vi "PIM Strip-Chart.vi"(4 "Clear Buffer (f)":bool, 5 "Buffer Length (2048)":i32=2048, 6 "Update Time, sec":dbl format="%.2f", 7 "Measured Values":dbl[](array[numeric])) -> (3 "Traces":cluster{"x-values":dbl[], "y-values":dbl[]}[](array[cluster]) {"y-values" format="%.2f"; "x-values" format="%.2f"})   [LabVIEW 2011]
doc: "Accepts a five element cluster of data points and buffers these into five separate clusters within an array (suitable for passing to an XY Chart).\n\nThe time, in Seconds since last reset, is placed in the x-value array for each line on the plot."
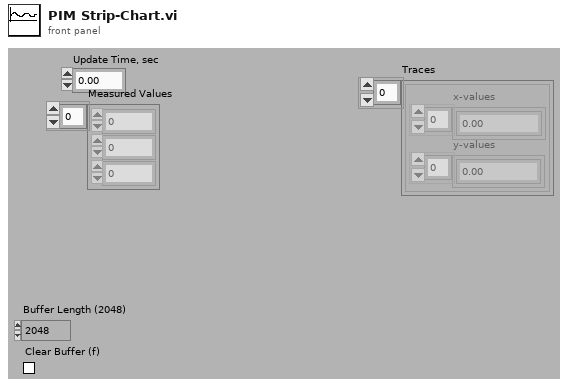
[diagram p1: front panel]
types:
  T1 = cluster{"Measured Values[0]":dbl, "Measured Values[1]":dbl}
  T2 = cluster{"Measured Values[0]":dbl, "Measured Values[1]":dbl, "Measured Values[2]":dbl, "Measured Values[3]":dbl, "Measured Values[4]":dbl}
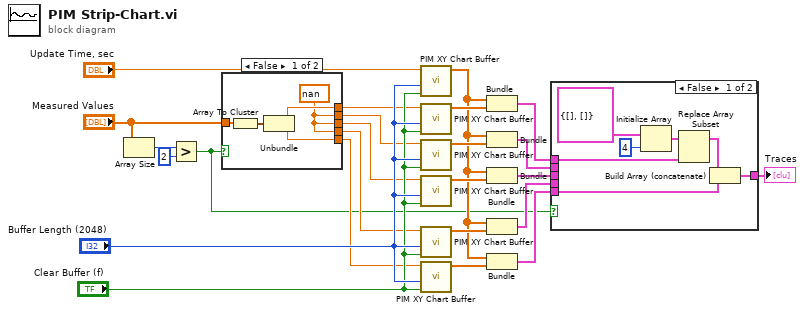
[diagram p0: block diagram]
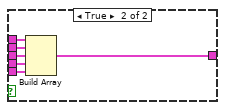
[diagram p2: hidden frame]
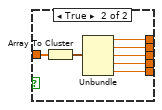
[diagram p3: hidden frame]
diagram:
  n1 = Array Size(array="Measured Values") -> (size(s)=w20:i32)
  n2 = Greater?(x=w20, y=2) -> (0:w1:bool)
  n3 = case shown="False" w1 {
    tunnel: "Measured Values" -> [w28 w36]
    tunnel: [w27 w35] -> w11
    tunnel: [w25 w34] -> w9
    tunnel: [w25 w33] -> w8
    tunnel: [w25 w32] -> w7
    tunnel: [w26 w31] -> w6
    frame False {
      w25 = nan ("Measured Values[3]")
      n4 = Array To Cluster(array=w28) -> (cluster=w29:T1)
      n5 = Unbundle(w29) -> ("Measured Values[0]"=w27:dbl, "Measured Values[1]"=w26:dbl)
    }
    frame True {
      n6 = Array To Cluster(array=w36) -> (cluster=w30:T2)
      n7 = Unbundle(w30) -> ("Measured Values[0]"=w35:dbl, "Measured Values[1]"=w34:dbl, "Measured Values[2]"=w33:dbl, "Measured Values[3]"=w32:dbl, "Measured Values[4]"=w31:dbl)
    }
  }
  n8 = call "PIM XY Chart Buffer.vi"("clear first (no:F)"="Clear Buffer (f)", "chart length (points)"="Buffer Length (2048)", "new number"="Update Time, sec") -> ("new array"=w2:dbl[])  [unwired: 1 in, 7 out]
  n9 = call "PIM XY Chart Buffer.vi"("clear first (no:F)"="Clear Buffer (f)", "chart length (points)"="Buffer Length (2048)", "new number"=w11) -> ("new array"=w10:dbl[])  [unwired: 1 in, 7 out]
  n10 = call "PIM XY Chart Buffer.vi"("clear first (no:F)"="Clear Buffer (f)", "chart length (points)"="Buffer Length (2048)", "new number"=w9) -> ("new array"=w12:dbl[])  [unwired: 1 in, 7 out]
  n11 = call "PIM XY Chart Buffer.vi"("clear first (no:F)"="Clear Buffer (f)", "chart length (points)"="Buffer Length (2048)", "new number"=w8) -> ("new array"=w3:dbl[])  [unwired: 1 in, 7 out]
  n12 = call "PIM XY Chart Buffer.vi"("clear first (no:F)"="Clear Buffer (f)", "chart length (points)"="Buffer Length (2048)", "new number"=w7) -> ("new array"=w4:dbl[])  [unwired: 1 in, 7 out]
  n13 = call "PIM XY Chart Buffer.vi"("clear first (no:F)"="Clear Buffer (f)", "chart length (points)"="Buffer Length (2048)", "new number"=w6) -> ("new array"=w5:dbl[])  [unwired: 1 in, 7 out]
  n14 = Bundle("new array"=w2, "new array"=w10) -> (w13:cluster{"new array":dbl[], "new array":dbl[]})  [unwired: 1 out]
  n15 = Bundle("new array"=w2, "new array"=w12) -> (w17:cluster{"new array":dbl[], "new array":dbl[]})  [unwired: 1 out]
  n16 = Bundle("new array"=w2, "new array"=w3) -> (w16:cluster{"new array":dbl[], "new array":dbl[]})  [unwired: 1 out]
  n17 = Bundle("new array"=w2, "new array"=w4) -> (w14:cluster{"new array":dbl[], "new array":dbl[]})  [unwired: 1 out]
  n18 = Bundle("new array"=w2, "new array"=w5) -> (w15:cluster{"new array":dbl[], "new array":dbl[]})  [unwired: 1 out]
  n19 = case shown="False" w1 {
    tunnel: [w43 w49] -> w23
    tunnel: w17 -> [_ w48]
    tunnel: w16 -> [_ w47]
    tunnel: w15 -> [w42 w46]
    tunnel: w14 -> [_ w45]
    tunnel: w13 -> [w38 w44]
    frame False {
      n20 = Initialize Array(cluster{dbl[], dbl[]} {[], []}, 4 ("dimension size")) -> (w41:cluster{dbl[], dbl[]}[])
      n21 = Replace Array Subset(array=w41, new element=w38) -> (w37:cluster{dbl[], dbl[]}[])  [unwired: 1 in]
      n22 = Build Array (concatenate)(w37, w42) -> (w43:cluster{"new array":dbl[], "new array":dbl[]}[])
    }
    frame True {
      n23 = Build Array(w44, w48, w47, w45, w46) -> (w49:cluster{"new array":dbl[], "new array":dbl[]}[])
    }
  }
  "Traces" <- w23
